vi "Log Level.vi"() -> ()   [LabVIEW 2020, in "CANopen Logging.lvlib"]
uses:
  CANopen Logging.lvlib
panel:
  in  "Log Level":T1(ring)
  # "1. ERROR\nOnly events that indicate a failure of the CANopen master or a node.  \nThis is the minimum level for production.\n\nLog when:\n\nNode goes to NMT state STOPPED/PRE-OP unexpectedly\n\nHeartbeat timeout or node guarding failure\n\nSDO abort codes (include index/subindex + abort reason)\n\nPDO mapping errors\n\nSYNC timing violations\n\nBus-off or CAN controller errors\n\nWhy: These events directly impact machine behavior and must be visible."
  # "2. WARN\nSuspicious or degraded conditions that don’t stop operation.\n\nLog when:\n\nNode recovers from heartbeat timeout\n\nSDO retries or slow responses\n\nPDO overrun/underrun detected\n\nUnexpected NMT transitions initiated by the node\n\nEMCY messages with non-critical error codes\n\nWhy: Helps detect flaky nodes or wiring issues before they become failures."
  # "3. INFO\nHigh-level operational events. Safe for production if rate-limited.\n\nLog when:\n\nMaster sends NMT commands (start/stop/reset)\n\nNode boots and sends boot-up message\n\nSYNC start/stop\n\nConfiguration steps (SDO writes during startup)\n\nEMCY messages (summarized)\n\nWhy: Useful for reconstructing system behavior without overwhelming logs."
  # "4. DEBUG\nDetailed protocol-level information. Usually disabled in production.\n\nLog when:\n\nAll SDO requests/responses\n\nPDO contents (decoded)\n\nSYNC timestamps\n\nLSS communication\n\nRaw CAN frames (filtered)\n\nWhy: Enables deep debugging but can overwhelm the bus and storage."
  # "5. TRACE\nExtremely verbose, frame-level tracing. Never enable in production.\n\nLog when:\n\nEvery CAN frame (RX/TX)\n\nTiming deltas between frames\n\nInternal state machine transitions\n\nWhy: Only for lab debugging or reproducing rare timing bugs."
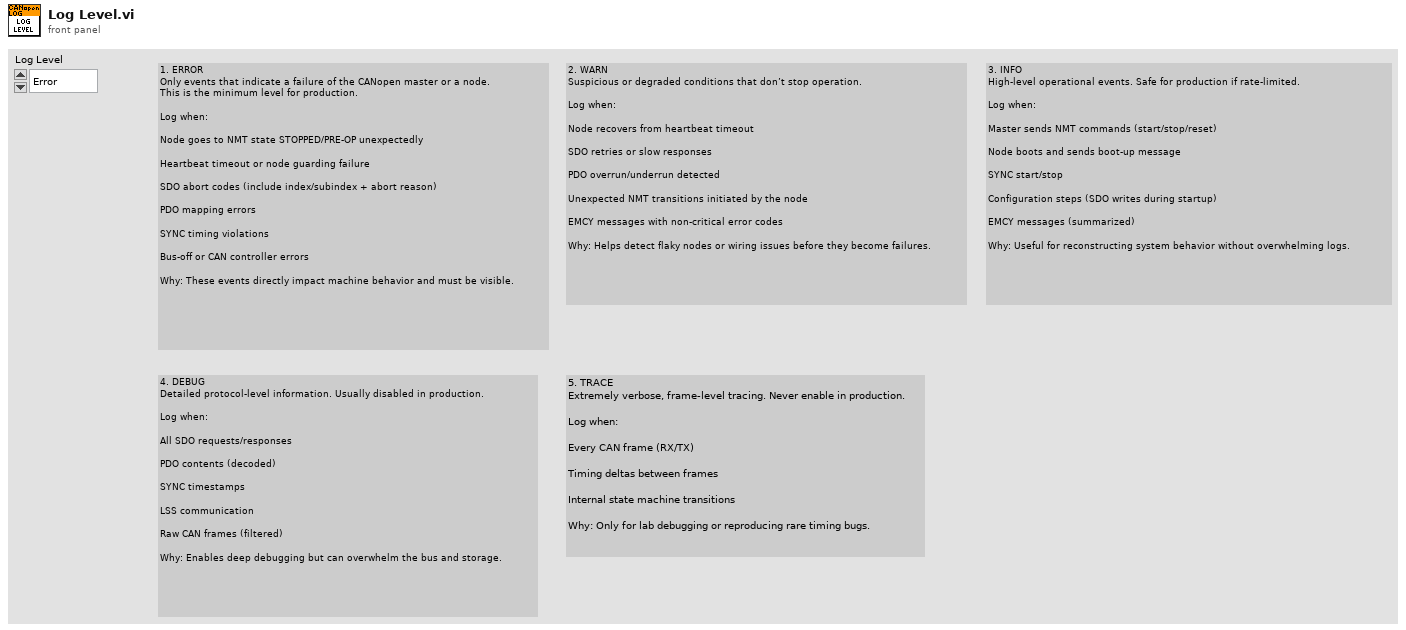
[diagram p1: front panel]
types:
  T1 = enum16{"Error", "Warn", "Info", "Debug", "Trace"}
diagram:
